vi "Get FIFO Command.vi"(11 "Neopixel Resources":T1={"Neopixel FIFO"="Neopixel FIFO", "Digital Output"="ConnectorC/DIO0"}) -> (2 "Timed Out?":bool, 3 "Command":T3)   [LabVIEW 2019, in "Neopixel - FPGA.lvlib"]
uses:
  Neopixel - FPGA.lvlib
  Shared/Public/Controls/Neopixel FIFO Command.ctl
  Public/Controls/Neopixel Resources.ctl
  Public/Controls/Neopixel FIFO.ctl
  <vilib>/rvi/DataTransferAndStorage/Container/Common/niFpgaContainerExecOnDevCompGetState.vi
  <vilib>/rvi/Emulation/niFpgaEmulationIsFPGAContextNoSignature.vi
  <vilib>/rvi/Emulation/niFpgaSctlEmulationGetInTimedLoop.vi
  <vilib>/rvi/errors/niFpgaSetErrorForExecOnDevCompSimple.vi
  <vilib>/rvi/eio/common/nirviEmuReportErrorAndStop.vi
  <vilib>/rvi/DataTransferAndStorage/Container/Common/niFpgaContainerGetUniqueNameForEmu.vi
  <vilib>/rvi/FIFO/Fifo_Resource/nirvififoEmulationSetSize.vi
  <vilib>/rvi/FIFO/Fifo_Resource/nirviFifoEmulationQueueMgr.vi
  <instcachedir>/0/nirviFifoEmulationQueueMgr_E5CAEC123FF24DC58D834DCA3CDAA9B5.lvgen/nirviFifoEmulationQueueMgr_E5CAEC123FF24DC58D834DCA3CDAA9B5_005.vi
  <vilib>/rvi/FIFO/Fifo_Resource/nirvififoEmulationDetermineInputValidOut.vi
  <vilib>/rvi/FIFO/Fifo_Resource/nirvififoEmulationCreateLock.vi
  <vilib>/rvi/Emulation/niFpgaProcessEmulError.vi
  <vilib>/rvi/FIFO/Fifo_Resource/nirvififoEmulationObtainLock.vi
  <vilib>/rvi/FIFO/Fifo_Resource/nirvififoEmulationReleaseLock.vi
  <vilib>/rvi/occurrence/nirviWaitOnOccurrenceBase.vi
  <vilib>/rvi/errors/nirviReportUnexpectedCaseInternalError.vi
  <vilib>/rvi/errors/nirviReportUnexpectedCaseInternalError (U32).vi
  <vilib>/Utility/error.llb/Clear Errors.vi
  <vilib>/rvi/interface/RandomDataEmulation/niFpgaRandomDataHandleErrors.vi
  <vilib>/rvi/DataTransferAndStorage/Container/XNode/niFpgaContainer.xnode
  <vilib>/rvi/FIFO/Fifo_Resource/niFpgaFifoEmulationRefIn.vi
  Shared/Neopixel Shared.lvlib
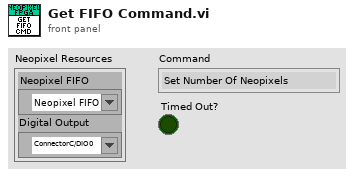
[diagram p1: front panel]
types:
  T1 = typedef "Neopixel - FPGA.lvlib/Neopixel Resources.ctl" = cluster{"Neopixel FIFO":T2, "Digital Output":refnum<k21>}
  T2 = typedef "Neopixel - FPGA.lvlib/Neopixel FIFO.ctl" = refnum<k21>
  T3 = typedef "Neopixel Shared.lvlib/Neopixel FIFO Command.ctl" = enum8{"Set Number Of Neopixels", "Update Frame"}
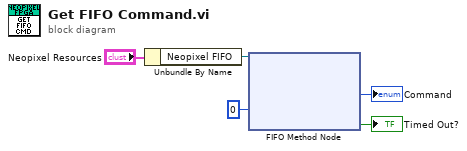
[diagram p0: block diagram]
diagram:
  n1 = Unbundle By Name("Neopixel Resources") -> ("Neopixel FIFO"=w1:T2)
  n2 = xnode ("FIFO Method Node")("Timeout"=0, "FIFO In"=w1) -> ("Element"=→"Command":u8, "Timed Out?"=→"Timed Out?":bool)  [unwired: 1 out]
